vi "Gait to K Lookup v2.vi"(11 "Current Gait %":dbl) -> (2 "Current K":dbl)   [LabVIEW 2018]
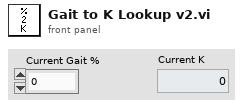
[diagram p1: front panel]
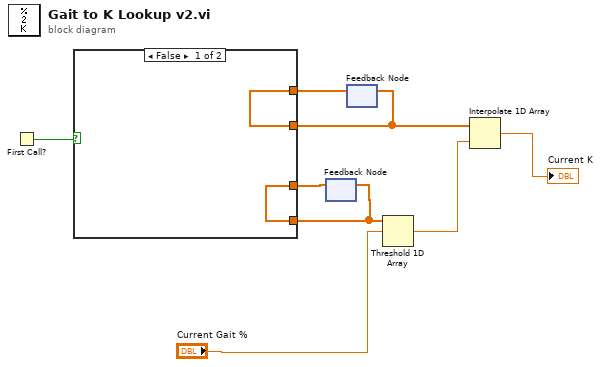
[diagram p0: block diagram]
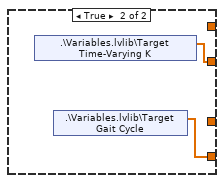
[diagram p2: hidden frame]
diagram:
  n1 = First Call?() -> (First Call?: T/F=w5:bool)
  n2 = feedback #1() -> (w2:dbl[])  [unwired: 1 in]
  n3 = feedback #2() -> (w1:dbl[])  [unwired: 1 in]
  n4 = case shown="False" w5 {
    tunnel: [w10 w12] -> w3
    tunnel: [w9 w11] -> w4
    tunnel: w2 -> [w10 _]
    tunnel: w1 -> [w9 _]
    frame False {
    }
    frame True {
      n5 = shared-variable ".\\Variables.lvlib\\Target Time-Varying K"() -> (w11:dbl[])  [unwired: 1 in, 1 out]
      n6 = shared-variable ".\\Variables.lvlib\\Target Gait Cycle"() -> (w12:dbl[])  [unwired: 1 in, 1 out]
    }
  }
  n7 = feedback-in #1(w3) -> ()
  n8 = feedback-in #2(w4) -> ()
  n9 = Threshold 1D Array(2:"Current Gait %", 3:w3) -> (0:w8:dbl)  [unwired: 1 in]
  n10 = Interpolate 1D Array(1:w8, 2:w4) -> (0:→"Current K":dbl)
